vi "Write Multiple Attributes.vi"(4 "Values":variant[](array[variant]), 5 "operation (open or create)":T1=enum."create or replace", 6 "error in (no error)":errorcluster, 8 "Names":string[](array[string]), 9 "HDF5 Ref":T2) -> (0 "error out":errorcluster, 3 "HDF5 Ref out":T2)   [LabVIEW 2017]
doc: "Writes multiple attributes to the specified HDF5 object"
uses:
  <vilib>/UPVI/lvhdf5/library.llb/HDF5 Ref.ctl
  <vilib>/UPVI/lvhdf5/attribute.llb/LVH5A Operation.ctl
panel:
  # "LVHDF5 Toolkit\nCopyright (c) 2005-2013 by Jason D. Sommerville\nCopyright (c) 2014 by UPVI, LLC.\n\nThis use and distribution of this file is governed by the terms found in \nLICENSE.txt distributed with this toolkit and installed at\n <user.lib>\\_lvhdf5\\LICENSE.txt"
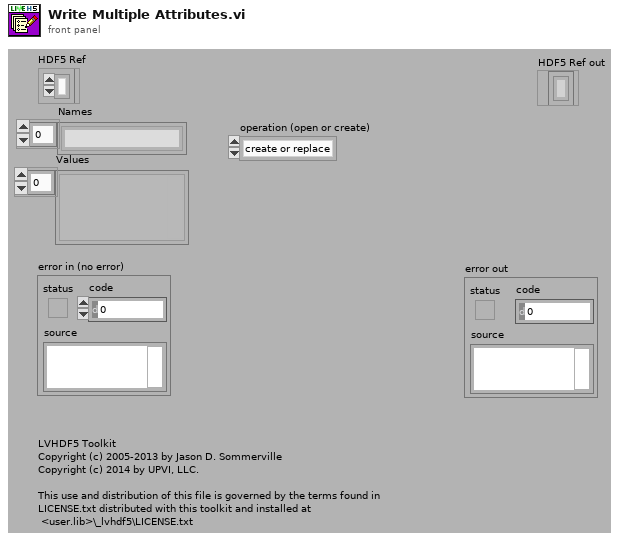
[diagram p1: front panel]
types:
  T1 = typedef "LVH5A Operation.ctl" = enum16{"open", "replace", "create", "open or create", "create or replace", "create or replace with confirmation"}
  T2 = typedef "HDF5 Ref.ctl" = refnum<k1>
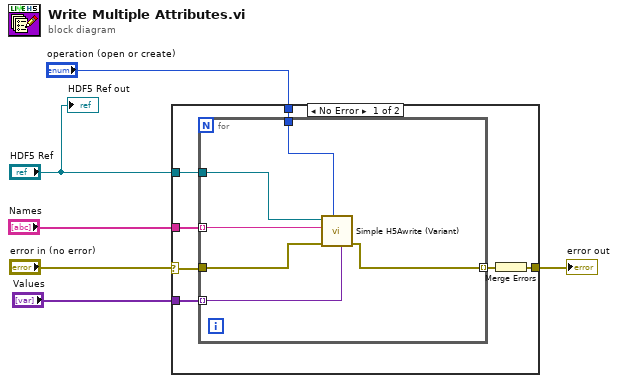
[diagram p0: block diagram]
diagram:
  n1 = case shown="No Error" "error in (no error)" {
    selector: "error in (no error)" -> [w9 w20]
    tunnel: "HDF5 Ref" -> [w13 _]
    tunnel: "Values" -> [w12 _]
    tunnel: "Names" -> [w11 _]
    tunnel: "operation (open or create)" -> [w10 _]
    tunnel: [w7 w20] -> w1
    frame No Error {
      n2 = for {
        tunnel: w13 -> [w19]
        tunnel: w12 -> [w16] mode=indexing
        tunnel: w11 -> [w18] mode=indexing
        tunnel: w10 -> [w17]
        tunnel: w9 -> [w15]
        tunnel: [w14] -> w8 mode=indexing
        n3 = call <vilib>:"Simple H5Awrite (Variant).vi"("Value"=w16, "operation (open or create)"=w17, "error in (no error)"=w15, "Name"=w18, "HDF5 Ref"=w19) -> ("error out"=w14:errorcluster)  [unwired: 3 in, 1 out]
      }
      n4 = Merge Errors(w8) -> (w7:errorcluster)
    }
    frame Error {
    }
  }
  "error out" <- w1
  "HDF5 Ref out" <- "HDF5 Ref"
